vi "fftnn.vi"() -> ()   [LabVIEW 2014]
doc: "This VI performs real-time Joint-Time Frequency Analysis (JTFA) using the STFT Spectrogram PtByPt VI. The signal is simulated by a sine wave plus Gaussian noise."
uses:
  <vilib>/DAQmx/create/channels.llb/DAQmx Create Channel (AI-Voltage-Basic).vi
  <vilib>/DAQmx/configure/timing.llb/DAQmx Timing (Sample Clock).vi
  <vilib>/DAQmx/read.llb/DAQmx Read (Analog DBL 1Chan 1Samp).vi
panel:
  in  "Sampling freq":dbl
  out "Intensity Graph":dbl[][](graph)
  in  "Halt!":bool
  out "in-loop read error":errorcluster
  out "daq create error":errorcluster
  out "timer create error":errorcluster
  in  "Fourier Transform size":i32(knob)=512 scale=4.0..512.0
  out "Now writing index...":i32=14
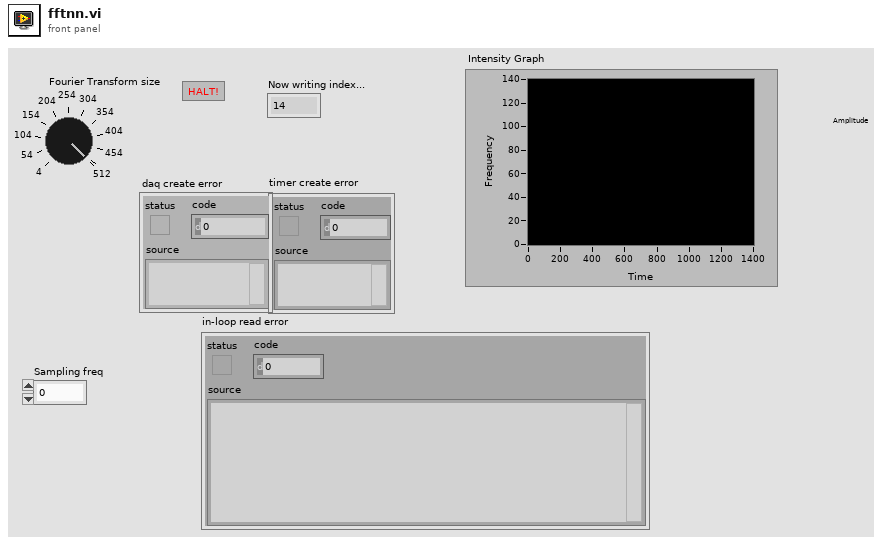
[diagram p1: front panel]
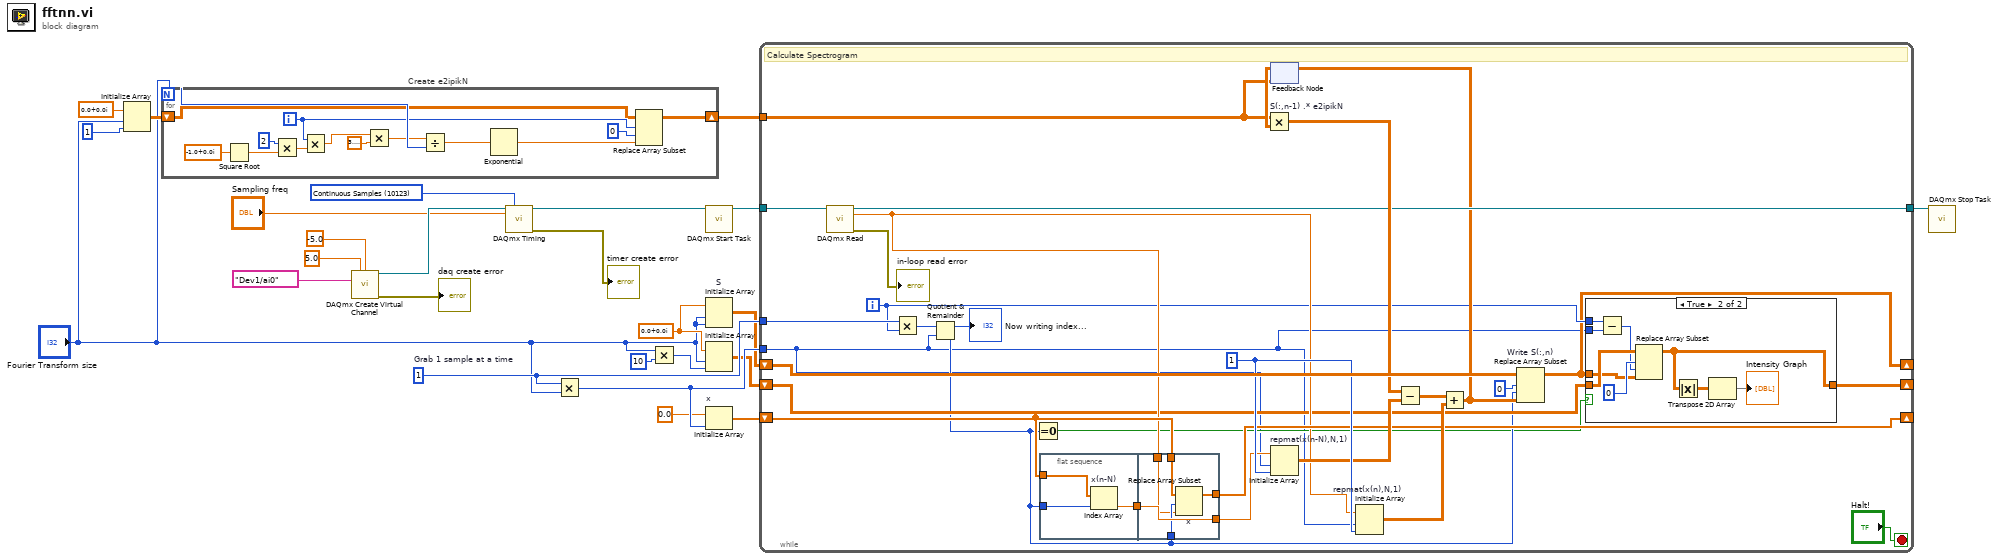
[diagram p0: block diagram]
diagram:
  w11 = 10123 items=["Finite Samples"=10178, "Continuous Samples"=10123, "Hardware Timed Single Point"=12522] ("sample mode")
  w6 = cdb 0.0+0.0i ("element")
  w22 = 1  # Grab 1 sample at a time
  n1 = Initialize Array(cdb 0.0+0.0i ("element"), "Fourier Transform size", 1 ("dimension size")) -> (w20:cdb[][])
  n2 = for "Create e2ipikN" {
    N: "Fourier Transform size" -> [w32]
    shift-right: [w30] -> w21
    shift-left: w20 -> [w28]
    i -> [w29]
    n3 = Square Root(x=cdb -1.0+0.0i) -> (sqrt(x)=w38:cdb)
    n4 = Multiply(x=2, y=w38) -> (x*y=w36:cdb)
    n5 = Multiply(x=w29, y=w36) -> (x*y=w35:cdb)
    n6 = Multiply(x=w35, y=3.141592653589793) -> (x*y=w31:cdb)
    n7 = Divide(x=w31, y=w32) -> (x/y=w33:cdb)
    n8 = Exponential(1:w33) -> (0:w26:cdb)
    n9 = Replace Array Subset(array=w28, new element=w26, index (row)=w29, index (col)=0 ("disabled index (col)")) -> (w30:cdb[][])
  }
  n10 = call-poly <vilib>:"DAQmx Create Virtual Channel.vi"("maximum value"=5.0, "minimum value"=-5.0, "physical channels"=tag "Dev1/ai0") -> ("task out"=w17:refnum<k21>, "error out"=→"daq create error":errorcluster)  [unwired: 11 in]
  n11 = call-poly <vilib>:"DAQmx Timing.vi"("task/channels in"=w17, "sample mode"=w11, "rate"="Sampling freq") -> ("task out"=w10:refnum<k21>, "error out"=→"timer create error":errorcluster)  [unwired: 11 in]
  n12 = Multiply(x=w22, y="Fourier Transform size") -> (x*y=w24:i32)
  n13 = Multiply(x="Fourier Transform size", y=10) -> (x*y=w4:i32)
  n14 = call <vilib>:"DAQmx Start Task.vi"("task/channels in"=w10) -> ("task out"=w8:refnum<k21>)  [unwired: 13 in, 1 out]
  n15 = Initialize Array "S"(w6, "Fourier Transform size", "Fourier Transform size") -> (w7:cdb[][])
  n16 = Initialize Array(w6, "Fourier Transform size", w4) -> (w5:cdb[][])
  n17 = Initialize Array "x"(0.0 ("element"), w24) -> (w25:dbl[])
  n18 = while {
    tunnel: w22 -> [w67]
    tunnel: w24 -> [w40]
    shift-right: [w51] -> _
    shift-left: w25 -> [w52]
    tunnel: w21 -> [w47]
    shift-right: [w43] -> _
    shift-left: w7 -> [w65]
    tunnel: w8 -> [w58]
    tunnel: [w57] -> w9
    shift-right: [w46] -> _
    shift-left: w5 -> [w45]
    i -> [w44]
    stop <- "Halt!" stop-if-true
    w63 = 1 ("dimension size")
    # "Calculate Spectrogram"
    n19 = call-poly <vilib>:"DAQmx Read.vi"("task/channels in"=w58) -> ("task out"=w57:refnum<k21>, "data"=w50:dbl, "error out"=→"in-loop read error":errorcluster)  [unwired: 12 in]
    n20 = Multiply(x=w67, y=w44) -> (x*y=w66:i32)
    n21 = Quotient & Remainder(x=w66, y=w40) -> (x-y*floor(x/y)=w42:i32)  [unwired: 1 out]
    "Now writing index..." <- w42
    n22 = Equal To 0?(x=w42) -> (x = 0?=w41:bool)
    n23 = flat-sequence {
      tunnel: w52 -> [w80]
      tunnel: w42 -> [w79]
      tunnel: [w78] -> w53
      tunnel: [w85] -> w54
      tunnel: w53 -> [w85]
      tunnel: w52 -> [w84]
      tunnel: [w83] -> w51
      tunnel: w42 -> [w82]
      tunnel: w50 -> [w81]
      frame #0 {
        n24 = Index Array "x(n-N)"(array=w80, index=w79) -> (element=w78:dbl)
      }
      frame #1 {
        n25 = Replace Array Subset "x"(array=w84, new element=w81, index=w82) -> (w83:dbl[])
      }
    }
    n26 = feedback #1(w47) -> (w48:cdb[][])
    n27 = Multiply "S(:,n-1) .* e2ipikN"(x=w47, y=w48) -> (x*y=w62:cdb[][])
    n28 = Initialize Array "repmat(x(n-N),N,1)"(w54, w40, w63) -> (w61:dbl[][])
    n29 = Initialize Array "repmat(x(n),N,1)"(w50, w40, w63) -> (w60:dbl[][])
    n30 = Subtract(x=w62, y=w61) -> (x-y=w59:cdb[][])
    n31 = Add(x=w59, y=w60) -> (x+y=w49:cdb[][])
    n32 = feedback-in #1(w49) -> ()
    n33 = Replace Array Subset "Write S(:,n)"(array=w65, new element=w49, index (row)=0, index (col)=w42) -> (w43:cdb[][])
    n34 = case shown="True" w41 {
      tunnel: [w68 w72] -> w46
      tunnel: w45 -> [w68 w77]
      tunnel: w44 -> [_ w71]
      tunnel: w43 -> [_ w75]
      tunnel: w40 -> [_ w70]
      frame False {
      }
      frame True {
        n35 = Subtract(x=w71, y=w70) -> (x-y=w69:i32)
        n36 = Replace Array Subset(array=w77, new element=w75, index (row)=0 ("disabled index (row)"), index (col)=w69) -> (w72:cdb[][])
        n37 = Absolute Value(x=w72) -> (abs(x)=w74:dbl[][])
        n38 = Transpose 2D Array(2D array=w74) -> (transposed array=→"Intensity Graph":dbl[][])
      }
    }
  }
  n39 = call <vilib>:"DAQmx Stop Task.vi"("task/channels in"=w9) -> ()  [unwired: 13 in, 2 out]
